vi "LED Matrix Anim TB.vi"() -> ()   [LabVIEW 2013]
uses:
  <vilib>/FPGAPlugInAG/myRIO-1900/niLvFpga_Open_myRIO-1900.vi
  <vilib>/rvi/interface/common/dynamic/niFpgaDynamicAddResources.vi
  <vilib>/myRIO/Common/Instrument Driver Framework/Utilities/vis/FPGA Ref Manager.vi
  <vilib>/Utility/error.llb/Error Cluster From Error Code.vi
  <vilib>/FPGAPlugInAG/Dynamic/niLvFpga_Close_Dynamic.vi
  <vilib>/rvi/interface/nirviOpenFPGA/nirviOpenFPGA.xnode
  FPGA Bitfiles/LEDMatrix4_FPGATarget_myRIO-1900Custom_r1aLzQW2H5E.lvbitx
  <vilib>/rvi/interface/nirviCloseFPGA/nirviCloseFPGA.xnode
  <vilib>/myRIO/Instrument Drivers/Utilities/Utilities.lvlib
panel:
  in  "stop":bool
  out "error out":errorcluster
  in  "rate (ms)":u32=100
  in  "Num FIles":i32=16
  in  "Brightness":u8=50 max=100 step=1
  in  "Factor":dbl=2.5
  out "LED Matrix":picture
  in  "path to BMP file on myRio local filesystem":path=path "/home/admin/images/pac_a.bmp"
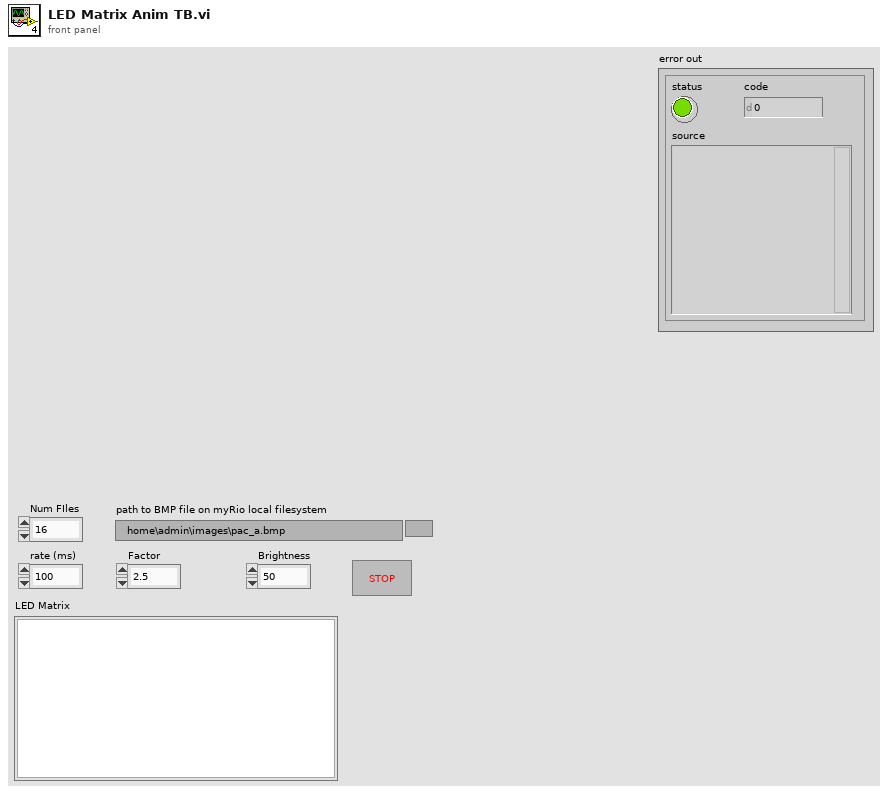
[diagram p1: front panel]
types:
  T1 = typedef "imagedata.ctl" = cluster{"image type":i32, "image depth":i32, "image":u8[], "mask":u8[], "colors":u32[], "Rectangle":cluster{"left":i16, "top":i16, "right":i16, "bottom":i16}}
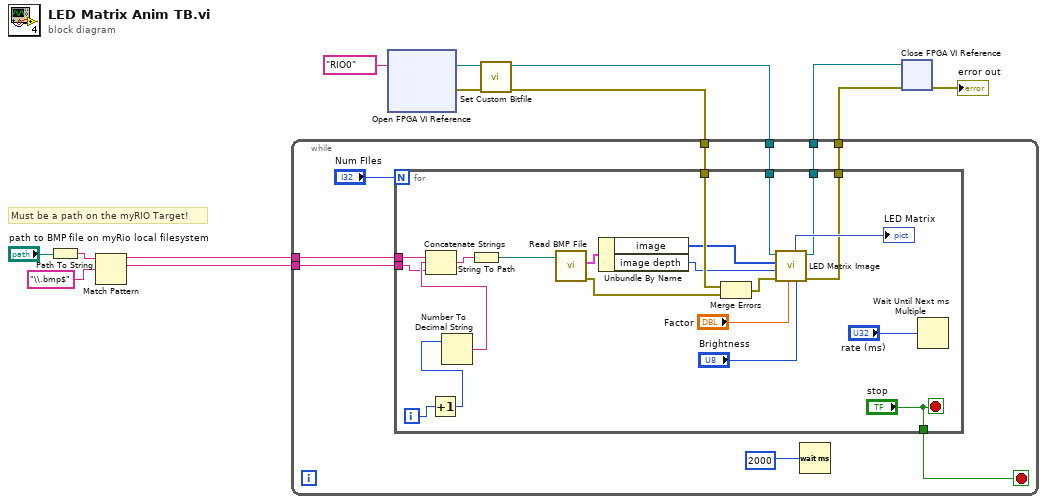
[diagram p0: block diagram]
diagram:
  # "Must be a path on the myRIO Target!"
  n1 = Path To String(path="path to BMP file on myRio local filesystem") -> (string=w12:string)
  n2 = Match Pattern(string=w12, regular expression="\\.bmp$") -> (before substring=w10:string, match substring=w9:string)  [unwired: 1 in, 2 out]
  n3 = xnode "Open FPGA VI Reference"("resource name"=tag "RIO0") -> ("FPGA VI Reference Out"=w7:refnum<k20>, "error out"=w6:errorcluster)  [unwired: 1 in]
  n4 = call <vilib>:"Set Custom Bitfile.vi"("error in (no error)"=w6, "Customized FPGA Reference in"=w7) -> ("error out"=w4:errorcluster, "Customized FPGA Reference out"=w5:refnum<k20>)  [unwired: 8 in]
  n5 = while {
    tunnel: w10 -> [w21]
    tunnel: w9 -> [w20]
    tunnel: w5 -> [w19]
    tunnel: w4 -> [w18]
    tunnel: [w17] -> w2
    tunnel: [w16] -> w1
    stop <- w15 stop-if-true
    n6 = for {
      N: "Num FIles" -> [_]
      tunnel: w21 -> [w42]
      tunnel: w20 -> [w40]
      tunnel: w19 -> [w28]
      tunnel: w18 -> [w30]
      tunnel: [w25] -> w17
      tunnel: [w24] -> w16
      tunnel: ["stop"] -> w15
      i -> [w36]
      stop <- "stop" stop-if-true
      n7 = Increment(x=w36) -> (x+1=w35:i32)
      n8 = Number To Decimal String(number=w35) -> (decimal integer string=w41:string)  [unwired: 1 in]
      n9 = Concatenate Strings(w42, w41, w40) -> (w39:string)
      n10 = String To Path(string=w39) -> (path=w38:path)
      n11 = call <vilib>:"Read BMP File.vi"("path to BMP file"=w38) -> ("error out"=w29:errorcluster, "image data"=w43:T1)  [unwired: 8 in, 1 out]
      n12 = Unbundle By Name(w43) -> ("image"=w26:u8[], "image depth"=w27:i32)
      n13 = Merge Errors(w30, w29) -> (w31:errorcluster)
      n14 = call "LED Matrix Image.vi"("Brightness"="Brightness", "Factor"="Factor", "error in (no error)"=w31, "image depth"=w27, "image"=w26, "Refnum in"=w28) -> ("error out"=w24:errorcluster, "Refnum out"=w25:refnum<k20>, "LED Matrix"=→"LED Matrix":picture)  [unwired: 3 in]
      n15 = Wait Until Next ms Multiple(millisecond multiple="rate (ms)") -> ()  [unwired: 1 out]
    }
    n16 = Wait (ms)(milliseconds to wait=u32 2000 ("millisecond multiple")) -> ()  [unwired: 1 out]
  }
  n17 = xnode "Close FPGA VI Reference"("FPGA VI Reference In"=w2, "error in"=w1) -> ("error out"=→"error out":errorcluster)
